vi "PFI-28000-System_Update Overloads.vi"(0 "PFI-28000-System in":refnum<class "PFI-28000-System.lvclass">, 5 "String":string, 11 "error in (no error)":errorcluster) -> (4 "PFI-28000-System out":refnum<class "PFI-28000-System.lvclass">, 15 "error out":errorcluster)   [LabVIEW 2017, in "PFI-28000-System.lvclass"]
uses:
  PFI-28000-System.lvclass
  C:/wc/07143 Precision Filters 28000 Support/Driver/source/Base/PFI-28000-Base.lvclass
  Overload/PFI-28000-Overload.lvclass
  <vilib>/regexp/Match Regular Expression.xnode
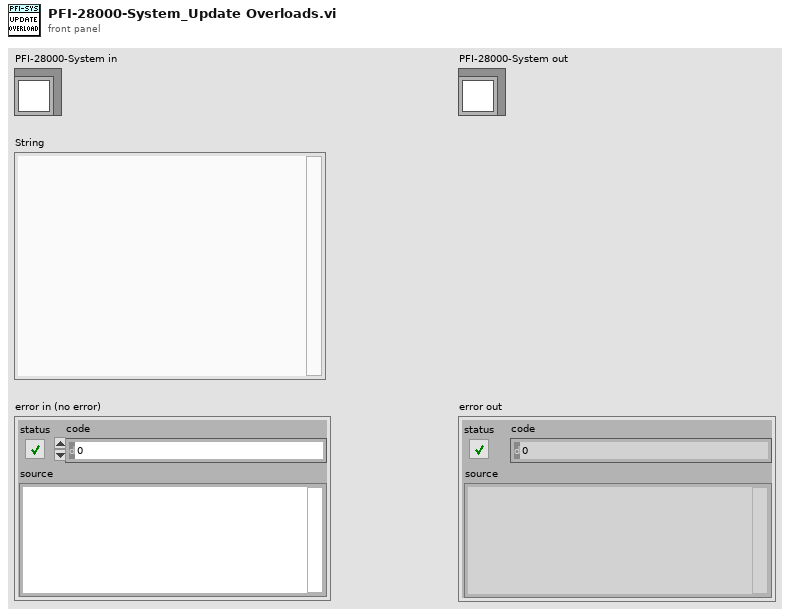
[diagram p1: front panel]
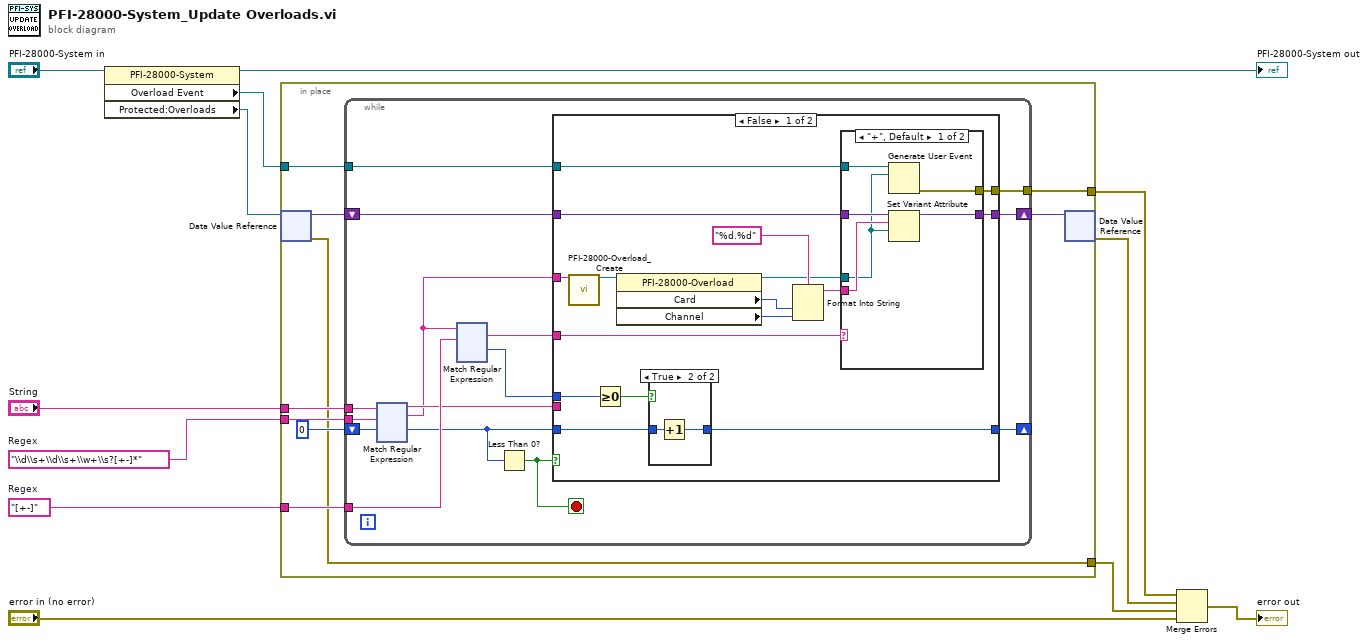
[diagram p0: block diagram]
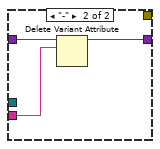
[diagram p3: hidden frame]
diagram:
  w6 = "[+-]"  # Regex
  w7 = "\\d\\s+\\d\\s+\\w+\\s?[+-]*"  # Regex
  n1 = property class="PFI-28000-System"(reference="PFI-28000-System in") -> (reference out=→"PFI-28000-System out":refnum<class "PFI-28000-System.lvclass">, "Overload Event"=w5:refnum<user-event>, "Protected:Overloads"=w9:refnum<data-value>)  [unwired: 1 in, 1 out]
  n2 = in-place {
    in-place-border: "String" -> [w20]
    in-place-border: w7 -> [w19]
    in-place-border: w6 -> [w17]
    in-place-border: w5 -> [w15]
    in-place-border: [w14] -> w1
    in-place-border: [w13] -> w3
    n3 = in-place-dvr #1(w9) -> (w21:variant, w13:errorcluster)
    n4 = while {
      tunnel: w20 -> [w36]
      tunnel: w19 -> [w35]
      shift-right: [w27] -> _
      shift-left: 0 ("offset past match") -> [w34]
      tunnel: w17 -> [w31]
      shift-right: [w32] -> w16
      shift-left: w21 -> [w33]
      tunnel: w15 -> [w23]
      tunnel: [w22] -> w14
      stop <- w29 stop-if-true
      n5 = xnode "Match Regular Expression"("input string"=w36, "regular expression"=w35, "offset (0)"=w34) -> ("before match"=w26:string, "whole match"=w25:string, "offset past match"=w24:i32)  [unwired: 3 in, 2 out]
      n6 = xnode "Match Regular Expression"("input string"=w25, "regular expression"=w31) -> ("whole match"=w30:string, "offset past match"=w28:i32)  [unwired: 4 in, 3 out]
      n7 = Less Than 0?(x=w24) -> (x < 0?=w29:bool)
      n8 = case shown="False" w29 {
        tunnel: w33 -> [w46 w66]
        tunnel: [w45 w66] -> w32
        tunnel: w25 -> [w44 _]
        tunnel: w30 -> [w43 _]
        tunnel: w28 -> [w42 _]
        tunnel: w24 -> [w40 w65]
        tunnel: [w39 w65] -> w27
        tunnel: w26 -> [_ _]
        tunnel: w23 -> [w38 _]
        tunnel: [w37 _] -> w22
        frame False {
          n9 = call "PFI-28000-Overload_Create.vi"("String"=w44) -> ("PFI-28000-Overload out"=w52:refnum<class "PFI-28000-Overload.lvclass">)  [unwired: 13 in, 1 out]
          n10 = Greater Or Equal To 0?(x=w42) -> (x >= 0?=w41:bool)
          n11 = property class="PFI-28000-Overload"(reference=w52) -> (reference out=w47:refnum<class "PFI-28000-Overload.lvclass">, "Card"=w51:i32, "Channel"=w50:i32)  [unwired: 1 in, 1 out]
          n12 = case shown="True" w41 {
            tunnel: w40 -> [w53 w55]
            tunnel: [w53 w54] -> w39
            frame False {
            }
            frame True {
              n13 = Increment(x=w55) -> (x+1=w54:i32)
            }
          }
          n14 = Format Into String(format string="%d.%d", w51, w50) -> (resulting string=w48:string)  [unwired: 2 in, 1 out]
          n15 = case shown="\"+\", Default" w43 {
            tunnel: w48 -> [w60 w63]
            tunnel: w47 -> [w57 _]
            tunnel: w46 -> [w61 w64]
            tunnel: [w59 w62] -> w45
            tunnel: w38 -> [w58 _]
            tunnel: [w56 _] -> w37
            frame "+", Default {
              n16 = Generate User Event(user event=w58, event data cluster=w57) -> (error out=w56:errorcluster)  [unwired: 2 in, 1 out]
              n17 = Set Variant Attribute(Variant=w61, name=w60, value=w57) -> (Variant out=w59:variant)  [unwired: 1 in, 2 out]
            }
            frame "-" {
              n18 = Delete Variant Attribute(6:w63, 7:w64) -> (3:w62:variant)  [unwired: 1 in, 2 out]
            }
          }
        }
        frame True {
        }
      }
    }
    n19 = in-place-dvr #1(w16) -> (w2:errorcluster)  [unwired: 1 out]
  }
  n20 = Merge Errors(w1, w2, w3, "error in (no error)") -> (→"error out":errorcluster)
